vi "floor types for qualification round.vi"(10 "cnt":i32, 11 "Type":enum16{"Z", "I", "O", "S", "L", "J", "T", "N"}(ring)) -> (3 "Type required":enum16{"Z", "I", "O", "S", "L", "J", "T", "N"}(ring))   [LabVIEW 2018]
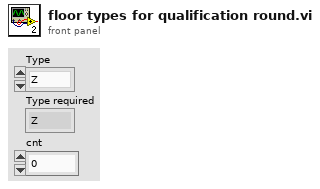
[diagram p1: front panel]
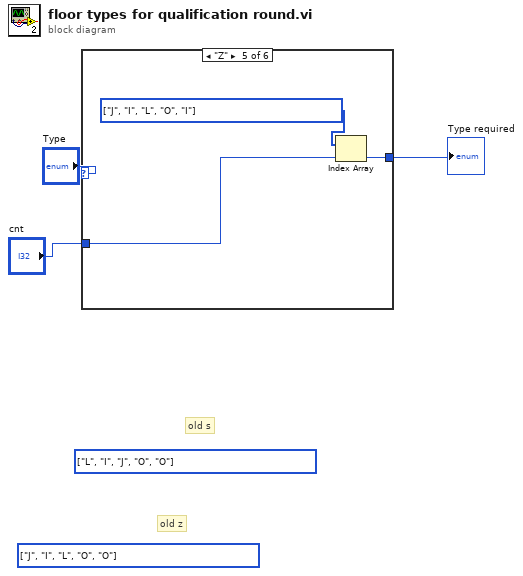
[diagram p0: block diagram]
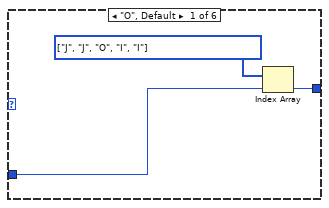
[diagram p2: hidden frame]
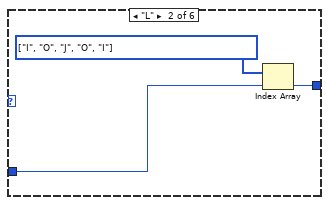
[diagram p3: hidden frame]
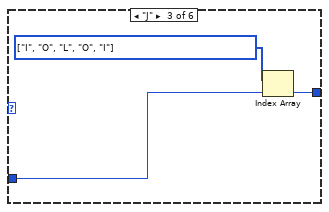
[diagram p4: hidden frame]
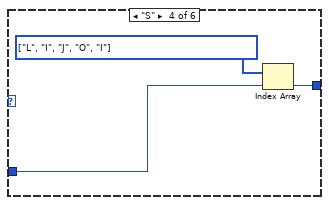
[diagram p5: hidden frame]
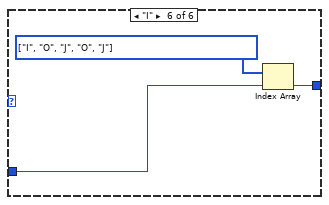
[diagram p6: hidden frame]
diagram:
  (unwired) enum16{"Z", "I", "O", "S", "L", "J", "T", "N"}[] [enum."J", enum."I", enum."L", enum."O", enum."O"] items=["Z", "I", "O", "S", "L", "J", "T", "N"] ("Type 2")
  (unwired) enum16{"Z", "I", "O", "S", "L", "J", "T", "N"}[] [enum."L", enum."I", enum."J", enum."O", enum."O"] items=["Z", "I", "O", "S", "L", "J", "T", "N"] ("Type 2")
  # "old z"
  # "old s"
  n1 = case shown="\"Z\"" "Type" {
    tunnel: "cnt" -> [w5 w8 w12 w14 w18 w20]
    tunnel: [w4 w7 w11 w13 w17 w19] -> w1
    frame "O", Default {
      w6 = enum16{"Z", "I", "O", "S", "L", "J", "T", "N"}[] [enum."J", enum."J", enum."O", enum."I", enum."I"] items=["Z", "I", "O", "S", "L", "J", "T", "N"] ("Type 2")
      n2 = Index Array(array=w6, index=w5) -> (element=w4:enum16{"Z", "I", "O", "S", "L", "J", "T", "N"})
    }
    frame "L" {
      w9 = enum16{"Z", "I", "O", "S", "L", "J", "T", "N"}[] [enum."I", enum."O", enum."J", enum."O", enum."I"] items=["Z", "I", "O", "S", "L", "J", "T", "N"] ("Type 2")
      n3 = Index Array(array=w9, index=w8) -> (element=w7:enum16{"Z", "I", "O", "S", "L", "J", "T", "N"})
    }
    frame "J" {
      w10 = enum16{"Z", "I", "O", "S", "L", "J", "T", "N"}[] [enum."I", enum."O", enum."L", enum."O", enum."I"] items=["Z", "I", "O", "S", "L", "J", "T", "N"] ("Type 2")
      n4 = Index Array(array=w10, index=w12) -> (element=w11:enum16{"Z", "I", "O", "S", "L", "J", "T", "N"})
    }
    frame "S" {
      w15 = enum16{"Z", "I", "O", "S", "L", "J", "T", "N"}[] [enum."L", enum."I", enum."J", enum."O", enum."I"] items=["Z", "I", "O", "S", "L", "J", "T", "N"] ("Type 2")
      n5 = Index Array(array=w15, index=w14) -> (element=w13:enum16{"Z", "I", "O", "S", "L", "J", "T", "N"})
    }
    frame "Z" {
      w16 = enum16{"Z", "I", "O", "S", "L", "J", "T", "N"}[] [enum."J", enum."I", enum."L", enum."O", enum."I"] items=["Z", "I", "O", "S", "L", "J", "T", "N"] ("Type 2")
      n6 = Index Array(array=w16, index=w18) -> (element=w17:enum16{"Z", "I", "O", "S", "L", "J", "T", "N"})
    }
    frame "I" {
      w21 = enum16{"Z", "I", "O", "S", "L", "J", "T", "N"}[] [enum."I", enum."O", enum."J", enum."O", enum."J"] items=["Z", "I", "O", "S", "L", "J", "T", "N"] ("Type 2")
      n7 = Index Array(array=w21, index=w20) -> (element=w19:enum16{"Z", "I", "O", "S", "L", "J", "T", "N"})
    }
  }
  "Type required" <- w1
